vi "Create Frame Pattern Script.vi"(8 "error in (no error)":errorcluster, 10 "SPI_FRM_Config":T1 {"Addr" format="%x"; "Data" format="%x"}, 11 "SPI_Frame_Read_Compare in":refnum<class "SPI_Frame_Read_Compare.lvclass">) -> (0 "error out":errorcluster, 3 "SPI_Frame_Read_Compare out":refnum<class "SPI_Frame_Read_Compare.lvclass">)   [LabVIEW 2018, in "SPI_Frame_Read_Compare.lvclass"]
uses:
  SPI_Frame_Read_Compare.lvclass
  C:/P4 Workspace/PC Client/Solutions/5g_eap/HiSi/trunk/1.0/BML_Pattern_Gen_Refactor/SPI/SPI Frame Root/SPI_Frame_Root.lvclass
  Config Read SPI/SPI_FRM_Config.ctl
  Classes/Config_Read/RW_Option.ctl
  Config Read SPI/SPI_Mode.ctl
  Classes/BML_Frame_Root/Special Frame.ctl
  SPI Frame Root/DataType.ctl
  SPI Frame Root/SPI_Frame_Root.lvclass/SPI_Frame_Root.ctl
  Classes/BML_Frame_Root/BML_Frame_Root.lvclass
  SPI Frame Root/SPI_Frame_Root.lvclass
  Classes/Config_Read/Config_Read_BML.lvclass
  Config Read SPI/Config_Read_SPI.lvclass
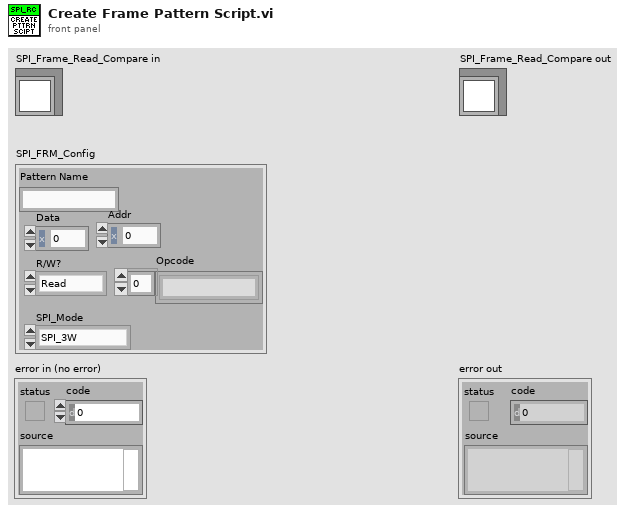
[diagram p1: front panel]
types:
  T1 = typedef "Config_Read_SPI.lvclass/SPI_FRM_Config.ctl" = cluster{"Pattern Name":string, "Data":u16, "Addr":u16, "R/W?":T2, "Opcode":string[], "SPI_Mode":T3}
  T2 = typedef "Config_Read_BML.lvclass/RW_Option.ctl" = enum16{"Read", "Write", "R/W"}
  T3 = typedef "Config_Read_SPI.lvclass/SPI_Mode.ctl" = enum16{"SPI_3W", "SPI_4W"}
  T4 = typedef "BML_Frame_Root.lvclass/Special Frame.ctl" = enum16{"Sync Header", "Protocol Header", "SW Trig", "SetID State", "Out SetID State", "SW Reset", "Wait", "SPI 4W FRM Start", "SPI 4W Wait", "SPI 4W FRM End", "SPI 4W Write Cmd", "SPI RD Collect Cmd", "SPI RD Value Cmd", "SPI 3W FRM Start", "SPI 3W Write Cmd", "SPI 3W FRM End", "SPI 3W Wait", "SPI 3W RD Cmd"}
  T5 = typedef "SPI_Frame_Root.lvclass/DataType.ctl" = enum16{"Drive", "Compare", "Read"}
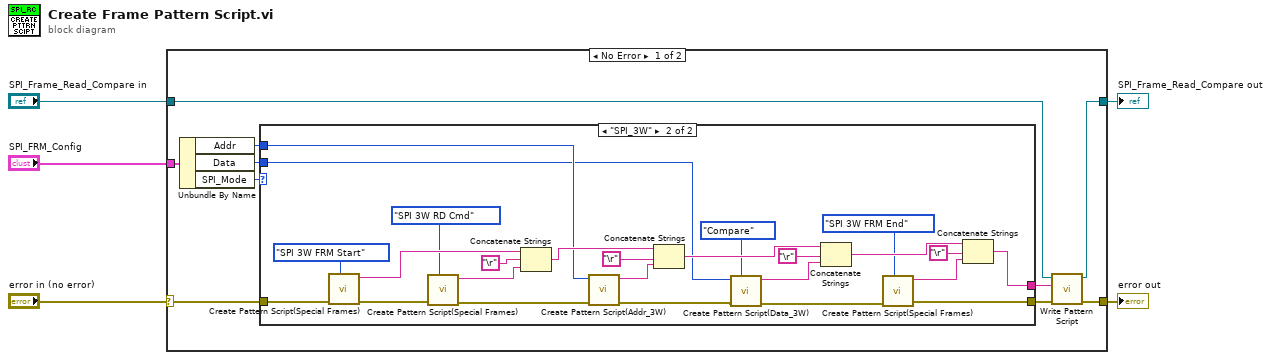
[diagram p0: block diagram]
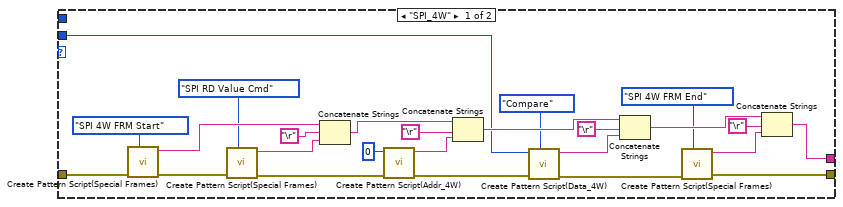
[diagram p2: hidden frame]
diagram:
  n1 = case shown="No Error" "error in (no error)" {
    selector: "error in (no error)" -> [w15 w67]
    tunnel: [w10 w67] -> w4
    tunnel: "SPI_Frame_Read_Compare in" -> [w9 w66]
    tunnel: [w8 w66] -> w2
    tunnel: "SPI_FRM_Config" -> [w14 _]
    frame No Error {
      n2 = Unbundle By Name(w14) -> ("Addr"=w6:u16, "Data"=w13:u16, "SPI_Mode"=w7:T3)
      n3 = case shown="\"SPI_3W\"" w7 {
        tunnel: w15 -> [w26 w56]
        tunnel: w13 -> [w25 w45]
        tunnel: [w20 w52] -> w12
        tunnel: [w19 w51] -> w11
        tunnel: w6 -> [_ w46]
        frame "SPI_4W" {
          n4 = call "Create Pattern Script(Special Frames).vi"("Special Frame Type"=Special_Frame."SPI 4W FRM Start", "error in (no error)"=w26) -> ("error out"=w27:errorcluster, "string out"=w29:string)  [unwired: 8 in]
          n5 = call "Create Pattern Script(Special Frames).vi"("Special Frame Type"=Special_Frame."SPI RD Value Cmd", "error in (no error)"=w27) -> ("error out"=w32:errorcluster, "string out"=w31:string)  [unwired: 8 in]
          n6 = Concatenate Strings(w29, "\r", w31) -> (w33:string)
          n7 = call "Create Pattern Script(Addr_4W).vi"("error in (no error)"=w32, "Addr"=u16 0) -> ("error out"=w36:errorcluster, "String"=w35:string)  [unwired: 8 in]
          n8 = Concatenate Strings(w33, "\r", w35) -> (w38:string)
          n9 = call "Create Pattern Script(Data_4W).vi"("DataType"=DataType."Compare", "error in (no error)"=w36, "Data"=w25) -> ("error out"=w24:errorcluster, "String"=w40:string)  [unwired: 7 in]
          n10 = Concatenate Strings(w38, "\r", w40) -> (w23:string)
          n11 = call "Create Pattern Script(Special Frames).vi"("Special Frame Type"=Special_Frame."SPI 4W FRM End", "error in (no error)"=w24) -> ("error out"=w20:errorcluster, "string out"=w21:string)  [unwired: 8 in]
          n12 = Concatenate Strings(w23, "\r", w21) -> (w19:string)
        }
        frame "SPI_3W" {
          n13 = call "Create Pattern Script(Special Frames).vi"("Special Frame Type"=Special_Frame."SPI 3W FRM Start", "error in (no error)"=w56) -> ("error out"=w57:errorcluster, "string out"=w59:string)  [unwired: 8 in]
          n14 = call "Create Pattern Script(Special Frames).vi"("Special Frame Type"=Special_Frame."SPI 3W RD Cmd", "error in (no error)"=w57) -> ("error out"=w47:errorcluster, "string out"=w61:string)  [unwired: 8 in]
          n15 = Concatenate Strings(w59, "\r", w61) -> (w62:string)
          n16 = call "Create Pattern Script(Addr_3W).vi"("error in (no error)"=w47, "Addr"=w46) -> ("error out"=w44:errorcluster, "String"=w48:string)  [unwired: 8 in]
          n17 = Concatenate Strings(w62, "\r", w48) -> (w64:string)
          n18 = call "Create Pattern Script(Data_3W).vi"("DataType"=DataType."Compare", "error in (no error)"=w44, "Data"=w45) -> ("error out"=w43:errorcluster, "String"=w42:string)  [unwired: 7 in]
          n19 = Concatenate Strings(w64, "\r", w42) -> (w55:string)
          n20 = call "Create Pattern Script(Special Frames).vi"("Special Frame Type"=Special_Frame."SPI 3W FRM End", "error in (no error)"=w43) -> ("error out"=w52:errorcluster, "string out"=w53:string)  [unwired: 8 in]
          n21 = Concatenate Strings(w55, "\r", w53) -> (w51:string)
        }
      }
      n22 = call "Write Pattern Script.vi"("error in (no error)"=w12, "Pattern Script"=w11, "SPI_Frame_Root in"=w9) -> ("error out"=w10:errorcluster, "SPI_Frame_Root out"=w8:refnum<class "SPI_Frame_Read_Compare.lvclass">)  [unwired: 7 in]
    }
    frame Error {
    }
  }
  "error out" <- w4
  "SPI_Frame_Read_Compare out" <- w2
